vi "InitFPGA.vi"() -> (0 "error out":errorcluster, 3 "Refnum out":refnum<k20>)   [LabVIEW 2019]
uses:
  <vilib>/userdefined/High Color/nirio_resource_hc.ctl
  <vilib>/FPGAPlugInAG/myRIO-1900/niLvFpga_Open_myRIO-1900.vi
  <vilib>/rvi/interface/common/dynamic/niFpgaDynamicAddResources.vi
  <vilib>/Utility/error.llb/Error Cluster From Error Code.vi
  <vilib>/rvi/errors/niLvFpgaAdjustHostInterfaceError.vi
  <vilib>/myRIO/Common/Instrument Driver Framework/Utilities/vis/FPGA Ref Manager.vi
  <vilib>/myRIO/Common/Instrument Driver Framework/Utilities/vis/Ref Counter.vi
  <vilib>/FPGAPlugInAG/Dynamic/niLvFpga_Run_Dynamic.vi
  <vilib>/rvi/interface/nirviOpenFPGA/nirviOpenFPGA.xnode
  autobike_FPGATarget_myRIO-1900Custom_zQgCF+RzkZg.lvbitx
  <vilib>/rvi/interface/nirviReadWriteControl/nirviReadWriteControl.xnode
  <vilib>/rvi/interface/nirviMethod/nirviMethod.xnode
  <vilib>/myRIO/Instrument Drivers/Utilities/Utilities.lvlib
  NiFpgaLv.dll
  <vilib>/rvi/interface/Simulation/niFpgaSimulationCallBeginRW.vi
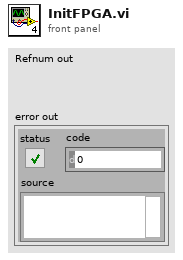
[diagram p1: front panel]
types:
  T1 = typedef "nirio_resource_hc.ctl" = tag
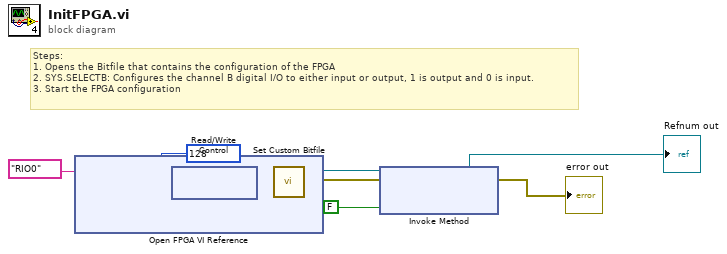
[diagram p0: block diagram]
diagram:
  # "Steps:\n1. Opens the Bitfile that contains the configuration of the FPGA\n2. SYS.SELECTB: Configures the channel B digital I/O to either input or output, 1 is output and 0 is input.\n3. Start the FPGA configuration"
  n1 = xnode "Open FPGA VI Reference"("resource name"=T1 "RIO0" ("Resource name")) -> ("FPGA VI Reference Out"=w8:refnum<k20>, "error out"=w9:errorcluster)  [unwired: 1 in]
  n2 = xnode "Read/Write Control"("FPGA VI Reference In"=w8, "error in"=w9, "SYS.SELECTB"=u8 128) -> ("FPGA VI Reference Out"=w4:refnum<k20>, "error out"=w5:errorcluster)
  n3 = call <vilib>:"Set Custom Bitfile.vi"("error in (no error)"=w5, "Custom FPGA Reference In"=w4) -> ("error out"=w3:errorcluster, "Custom FPGA Reference Out"=w1:refnum<k20>)  [unwired: 8 in]
  n4 = xnode "Invoke Method"("FPGA VI Reference In"=w1, "error in"=w3, "Wait Until Done (F)"=FALSE) -> ("FPGA VI Reference Out"=→"Refnum out":refnum<k20>, "error out"=→"error out":errorcluster)
